vi "host.vi"() -> ()   [LabVIEW 2020]
uses:
  <vilib>/Analysis/baseanly.llb/Real A x B.vi
  <vilib>/Analysis/baseanly.llb/Mean (DBL).vi
  <vilib>/Analysis/Matrix/Numeric/Conversions/Array To Matrix - RA2.vi
  <vilib>/Analysis/Matrix/Numeric/Conversions/Matrix To Array - RM.vi
  <vilib>/Analysis/7linalg.llb/Real Eigenvalues and Vectors.vi
  <vilib>/rvi/interface/RandomDataEmulation/nirviRandomDataOpen.vi
  <vilib>/rvi/interface/common/niFpgaCacheSessionInfoDynamic.vi
  <vilib>/Utility/error.llb/Error Cluster From Error Code.vi
  <vilib>/rvi/errors/niLvFpgaAdjustHostInterfaceError.vi
  <vilib>/FPGAPlugInAG/Dynamic/niLvFpga_Run_Dynamic.vi
  <vilib>/FPGAPlugInAG/Dynamic/niLvFpga_Close_Dynamic.vi
  <vilib>/rvi/interface/nirviOpenFPGA/nirviOpenFPGA.xnode
  target.vi
  <vilib>/rvi/interface/nirviMethod/nirviMethod.xnode
  <vilib>/rvi/interface/nirviCloseFPGA/nirviCloseFPGA.xnode
  <vilib>/rvi/errors/niLvFpgaMergeErrorWithErrorCode.vi
  <vilib>/Analysis/Matrix/NI_Matrix.lvlib
  <vilib>/Analysis/NI_AALBase.lvlib
  <vilib>/Analysis/NI_AALPro.lvlib
  <vilib>/FPGAPlugInAG/Dynamic/niLvFpga_WriteFifo_Dynamic.vi
  <vilib>/FPGAPlugInAG/Dynamic/niLvFpga_ReadFifo_Dynamic.vi
panel:
  out "A":dbl[][](array[numeric])
  out "LabVIEW eigvals":dbl[](array[numeric])
  out "FPGA Jacobi eigenvalue":sgl[](array[numeric])
  out "percent error":dbl
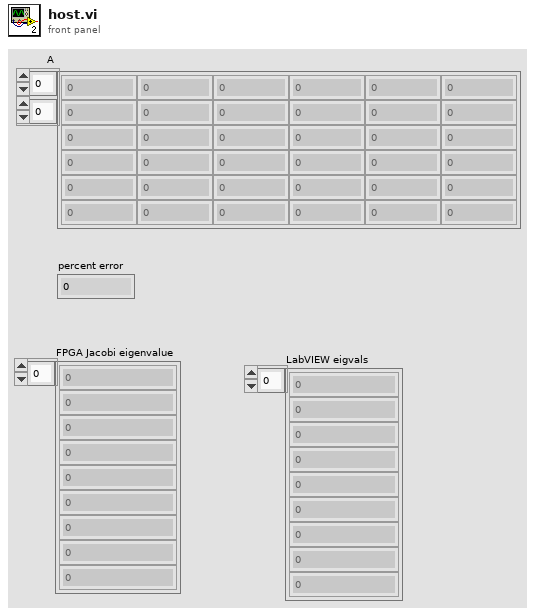
[diagram p1: front panel]
types:
  T1 = typedef "NI_Matrix.lvlib/RealMatrix.ctl" = dbl[][]
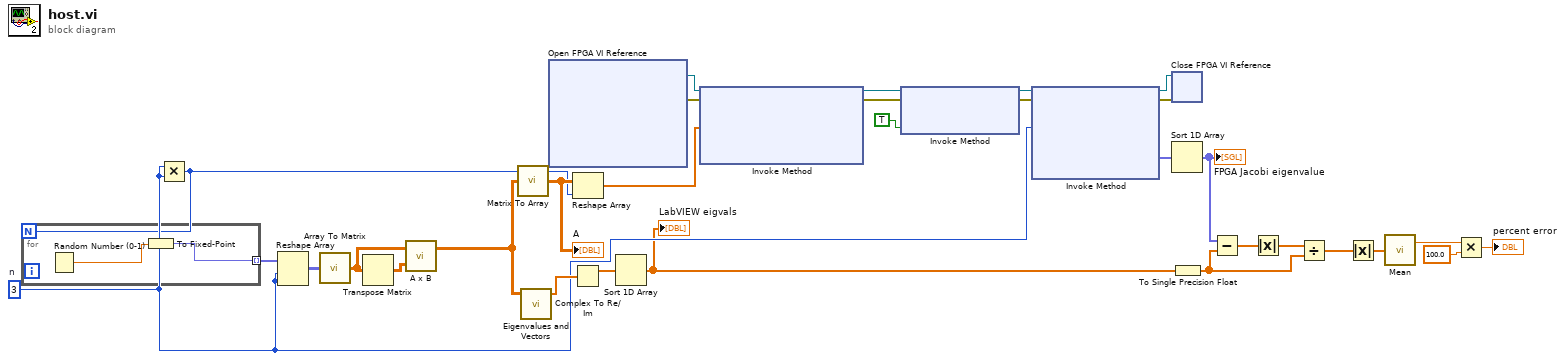
[diagram p0: block diagram]
diagram:
  w19 = 3  # n
  n1 = Multiply(x=w19, y=w19) -> (x*y=w14:i32)
  n2 = for {
    N: w14 -> [_]
    tunnel: [w32] -> w18 mode=indexing
    n3 = Random Number (0-1)() -> (number: 0 to 1=w33:dbl)
    n4 = To Fixed-Point(number=w33) -> (fixed-point=w32:fxp<+/-,32,16>)  [unwired: 1 in]
  }
  n5 = Reshape Array(w18, w19, w19) -> (w17:fxp<+/-,32,16>[][])
  n6 = call-poly <vilib>:"Array To Matrix.vi"("Real 2D Array"=w17) -> ("Real Matrix"=w16:T1)
  n7 = Transpose Matrix(1:w16) -> (0:w15:T1)
  n8 = call-poly <vilib>:"A x B.vi"("B"=w15, "A"=w16) -> ("A x B"=w23:T1)  [unwired: 1 out]
  n9 = call-poly <vilib>:"Matrix To Array.vi"("Real Matrix"=w23) -> ("Real 2D Array"=w21:dbl[][])
  "A" <- w21
  n10 = call-poly <vilib>:"Eigenvalues and Vectors.vi"("Input Matrix"=w23) -> ("Eigenvalues"=w24:cdb[])  [unwired: 2 in, 2 out]
  n11 = xnode "Open FPGA VI Reference"() -> ("FPGA VI Reference Out"=w30:refnum<k20>, "error out"=w29:errorcluster)  [unwired: 2 in]
  n12 = Reshape Array(w21, w14) -> (w1:dbl[])
  n13 = Complex To Re/Im(x + iy=w24) -> (x=w22:dbl[])  [unwired: 1 out]
  n14 = Sort 1D Array(array=w22) -> (sorted array=w13:dbl[])
  "LabVIEW eigvals" <- w13
  n15 = xnode "Invoke Method"("FPGA VI Reference In"=w30, "error in"=w29, "Data"=w1) -> ("FPGA VI Reference Out"=w26:refnum<k20>, "error out"=w25:errorcluster)  [unwired: 1 in, 1 out]
  n16 = xnode "Invoke Method"("FPGA VI Reference In"=w26, "error in"=w25, "Wait Until Done (F)"=TRUE) -> ("FPGA VI Reference Out"=w28:refnum<k20>, "error out"=w27:errorcluster)
  n17 = xnode "Invoke Method"("FPGA VI Reference In"=w28, "error in"=w27, "Number of Elements"=w19) -> ("FPGA VI Reference Out"=w3:refnum<k20>, "error out"=w2:errorcluster, "Data"=w20:fxp<+/-,32,16>[])  [unwired: 1 in, 1 out]
  n18 = xnode "Close FPGA VI Reference"("FPGA VI Reference In"=w3, "error in"=w2) -> ()  [unwired: 1 out]
  n19 = Sort 1D Array(array=w20) -> (sorted array=w12:fxp<+/-,32,16>[])
  "FPGA Jacobi eigenvalue" <- w12
  n20 = To Single Precision Float(number=w13) -> (single precision float=w9:sgl[])
  n21 = Subtract(x=w12, y=w9) -> (x-y=w11:sgl[])
  n22 = Absolute Value(x=w11) -> (abs(x)=w10:sgl[])
  n23 = Divide(x=w10, y=w9) -> (x/y=w8:sgl[])
  n24 = Absolute Value(x=w8) -> (abs(x)=w7:sgl[])
  n25 = call-poly <vilib>:"Mean.vi"("X"=w7) -> ("mean"=w6:dbl)  [unwired: 1 out]
  n26 = Multiply(x=w6, y=100.0) -> (x*y=→"percent error":dbl)
